vi "Read Source.vi"(8 "Error In":errorcluster, 11 "Node In":refnum<class "Partial.lvclass">) -> (0 "Error Out":errorcluster, 2 "Source":string, 3 "Node Out":refnum<class "Partial.lvclass">)   [LabVIEW 2018, in "Toolkit.lvlib" / "Nodes.lvlib" / "Partial.lvclass"]
doc: "Gets the original, raw text from the Mustache template that yielded the node during the parsing process.\n\n<B>Node In/Out</B> - Represents a node in the Abstract Syntax Tree (AST) of a parsed Mustache template.\n\n<B>Source</B> - The original, raw text from the Mustache template."
uses:
  Partial.lvclass
  Partial.lvclass/Partial.ctl
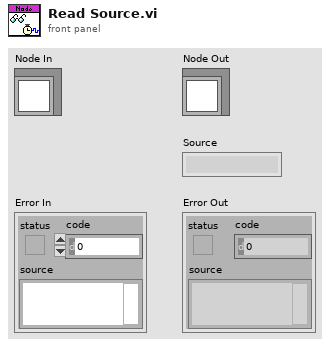
[diagram p1: front panel]
types:
  T1 = typedef "Toolkit.lvlib/Delimiters.ctl" = cluster{"Close":string, "Open":string}
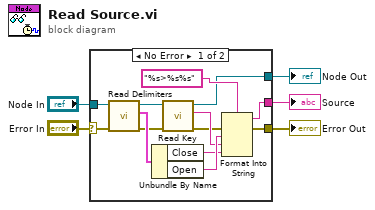
[diagram p0: block diagram]
diagram:
  n1 = case shown="No Error" "Error In" {
    selector: "Error In" -> [w17 w20]
    tunnel: [w9 w20] -> w4
    tunnel: "Node In" -> [w16 w19]
    tunnel: [w6 w19] -> w2
    tunnel: [w7 _] -> w1
    frame No Error {
      n2 = call-dynamic "Read Delimiters.vi"("Error In"=w17, "Node In"=w16) -> ("Error Out"=w12:errorcluster, "Delimiters"=w15:T1, "Node Out"=w13:refnum<class "Partial.lvclass">)  [unwired: 7 in]
      n3 = Unbundle By Name(w15) -> ("Close"=w8:string, "Open"=w14:string)
      n4 = call "Read Key.vi"("Error In"=w12, "Partial In"=w13) -> ("Error Out"=w10:errorcluster, "Key"=w11:string, "Partial Out"=w6:refnum<class "Partial.lvclass">)  [unwired: 7 in]
      n5 = Format Into String(format string="%s>%s%s", error in=w10, w14, w11, w8) -> (resulting string=w7:string, error out=w9:errorcluster)  [unwired: 1 in]
    }
    frame Error {
    }
  }
  "Error Out" <- w4
  "Node Out" <- w2
  "Source" <- w1
